vi "(SubVI) Deal with Delay between Scan and Record From Stage Array-v2.vi"(4 "Avg. time delay (ms)":dbl=18.0, 5 "Toward first ?\nT=+, F=-":bool, 6 "Record scan rate  (um/s)":dbl=2.0 format="%.3f", 7 "Real initial position (um)":dbl format="%0.5f", 8 "Folded Stage Array (um)":dbl[](array[numeric]), 9 "Unfolded Stage Array (um)":dbl[](array[numeric])) -> (0 "Stage Array Shift (nm)":dbl, 2 "Correct Folded Stage Array (um)":dbl[](array[numeric]), 3 "Correct Unfolded Stage Array (um)":dbl[](array[numeric]))   [LabVIEW 2014]
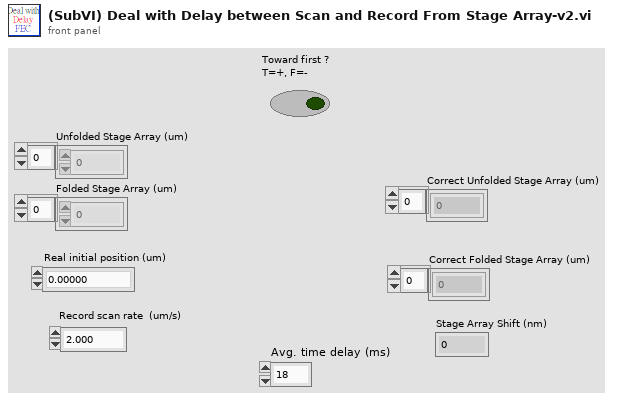
[diagram p1: front panel]
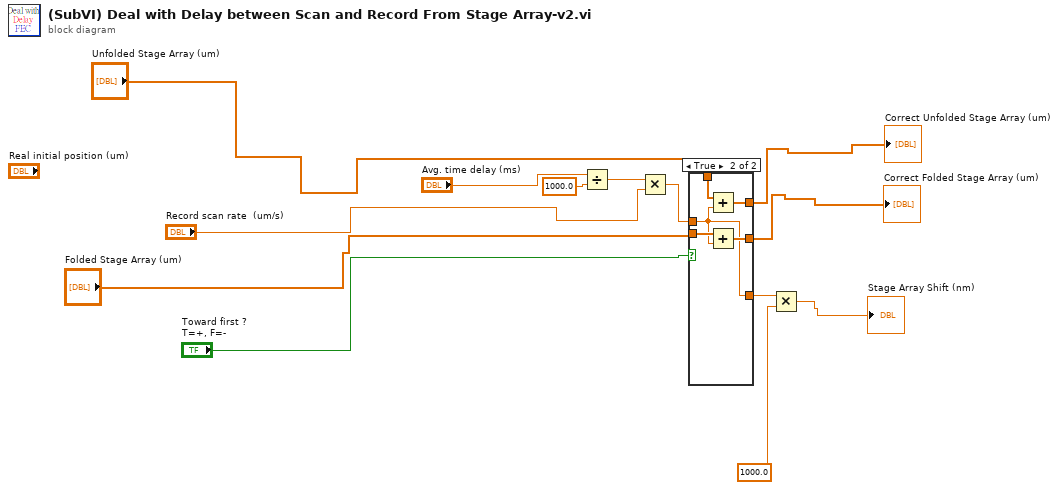
[diagram p0: block diagram]
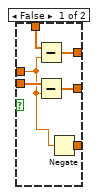
[diagram p2: hidden frame]
diagram:
  n1 = Divide(x="Avg. time delay (ms)", y=1000.0) -> (x/y=w8:dbl)
  n2 = Multiply(x=w8, y="Record scan rate  (um/s)") -> (x*y=w10:dbl)
  n3 = case shown="True" "Toward first ?\nT=+, F=-" {
    tunnel: "Folded Stage Array (um)" -> [w19 w24]
    tunnel: w10 -> [w16 w21]
    tunnel: [w18 w23] -> w2
    tunnel: [w17 w22] -> w1
    tunnel: [w15 w21] -> w6
    tunnel: "Unfolded Stage Array (um)" -> [w14 w20]
    frame False {
      n4 = Subtract(x=w14, y=w16) -> (x-y=w17:dbl[])
      n5 = Subtract(x=w19, y=w16) -> (x-y=w18:dbl[])
      n6 = Negate(x=w16) -> (-x=w15:dbl)
    }
    frame True {
      n7 = Add(x=w20, y=w21) -> (x+y=w22:dbl[])
      n8 = Add(x=w24, y=w21) -> (x+y=w23:dbl[])
    }
  }
  "Correct Unfolded Stage Array (um)" <- w1
  "Correct Folded Stage Array (um)" <- w2
  n9 = Multiply(x=w6, y=1000.0) -> (x*y=→"Stage Array Shift (nm)":dbl)
